vi "Config - Update Data.vi"(8 "error in (no error)":errorcluster, 11 "Config Data":T1 {"Step Duration" max=99999 step=1}) -> (0 "error out":errorcluster, 3 "Config Data":T1 {"Step Duration" max=99999 step=1})   [LabVIEW 2017]
doc: "Provide update data records in the XML file"
uses:
  Controls/Congif Data.ctl
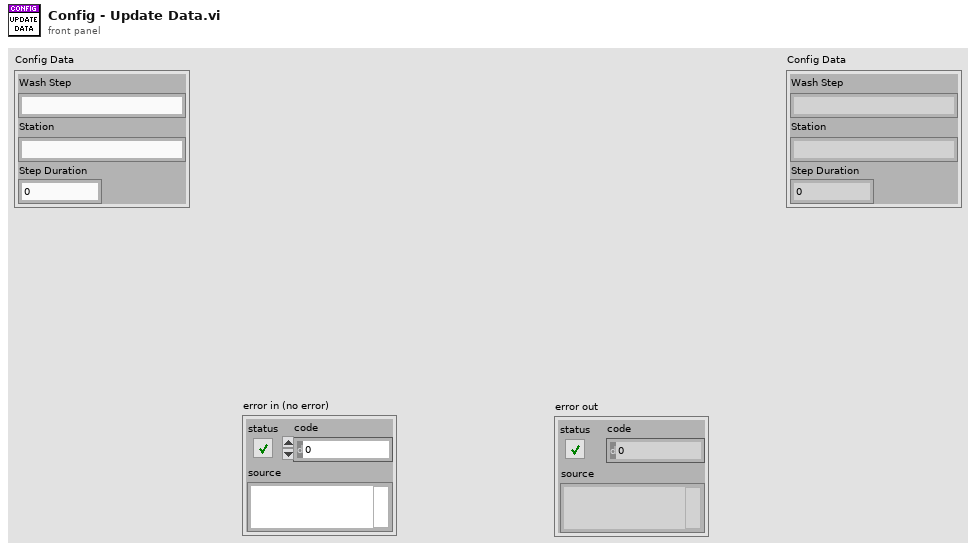
[diagram p1: front panel]
types:
  T1 = typedef "Congif Data.ctl" = cluster{"Wash Step":string, "Station":string, "Step Duration":u32}
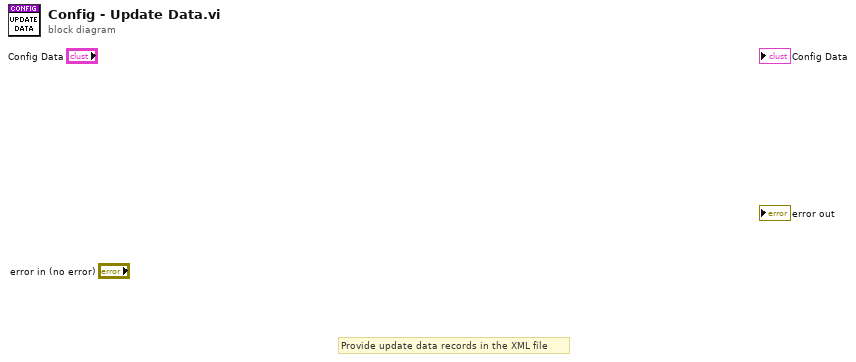
[diagram p0: block diagram]
diagram:
  # "Provide update data records in the XML file"
